vi "Write configuration.vi"(8 "error in (no error)":errorcluster, 10 "configuration":refnum<class "CEF_serializable configuration.lvclass">, 11 "Fgen Instrument":refnum<class "Fgen Instrument.lvclass">) -> (0 "error out":errorcluster, 3 "Fgen Instrument out":refnum<class "Fgen Instrument.lvclass">)   [LabVIEW 2025, in "Fgen.lvlib" / "Fgen Instrument.lvclass"]
uses:
  Fgen Instrument.lvclass
  Users/Public/Documents/Sandia National Labs/TSS Plugin/CEF.lvlibp/serializable configuration/CEF_serializable configuration.lvclass
  Fgen configuration/Fgen configuration.lvclass
  Fgen Instrument.lvclass/Fgen Instrument.ctl
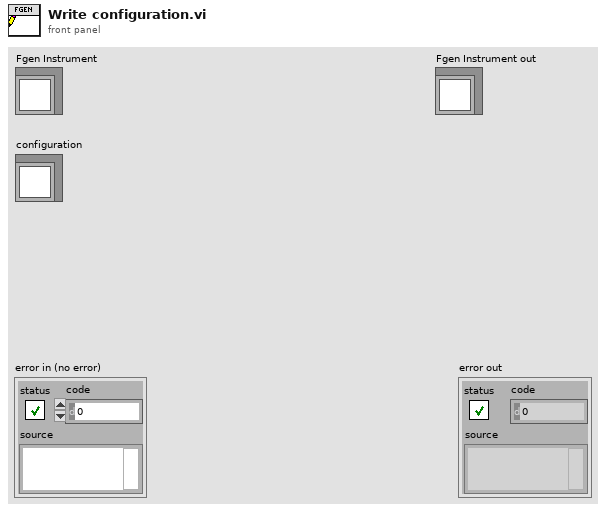
[diagram p1: front panel]
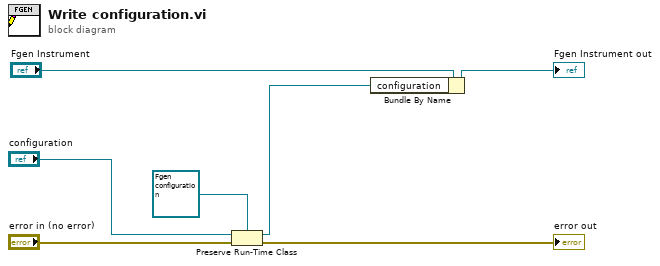
[diagram p0: block diagram]
diagram:
  n1 = Preserve Run-Time Class(object in="configuration", error in="error in (no error)", 2:refnum<class "Fgen configuration.lvclass"> refnum ("Fgen.lvlib:Fgen configuration.lvclass")) -> (object out=w4:refnum<class "Fgen configuration.lvclass">, error out=→"error out":errorcluster)
  n2 = Bundle By Name(cluster="Fgen Instrument", "configuration"=w4) -> (→"Fgen Instrument out":refnum<class "Fgen Instrument.lvclass">)
